vi "initialize ASI stage.vi"(4 "set pcros (um)":cluster{"X":dbl, "Y":dbl, "Z":dbl}, 5 "y range":dbl, 6 "z range":dbl, 7 "x range":dbl, 8 "error in (no error)":errorcluster, 9 "timeout":u32=100, 10 "Baud rate":u32=115200, 11 "VISA resource name":refnum<visa-resource-name>) -> (0 "error out":errorcluster, 3 "ASI stage":T1)   [LabVIEW 2010]
uses:
  stage properties.ctl
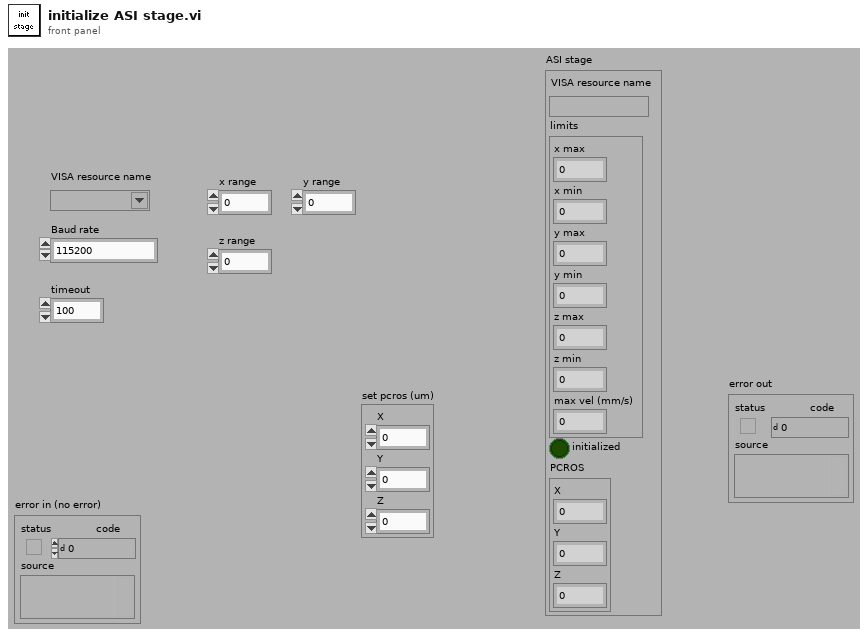
[diagram p1: front panel]
types:
  T1 = typedef "stage properties.ctl" = cluster{"VISA resource name":refnum<visa-resource-name>, "limits":cluster{"x max":dbl, "x min":dbl, "y max":dbl, "y min":dbl, "z max":dbl, "z min":dbl, "max vel (mm/s)":dbl}, "initialized":bool, "PCROS":cluster{"X":dbl, "Y":dbl, "Z":dbl}}
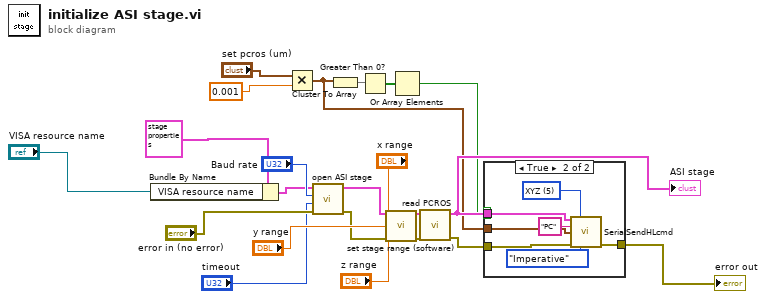
[diagram p0: block diagram]
diagram:
  n1 = Bundle By Name(cluster=T1 {"VISA resource name"="", "limits"={"x max"=0.0, "x min"=0.0, "y max"=0.0, "y min"=0.0, "z max"=0.0, "z min"=0.0, "max vel (mm/s)"=0.0}, "initialized"=FALSE, "PCROS"={"X"=0.0, "Y"=0.0, "Z"=0.0}} ("ASI stage"), "VISA resource name"="VISA resource name") -> (w14:T1)
  n2 = Multiply(x="set pcros (um)", y=0.001 ("x range")) -> (x*y=w5:cluster{"X":dbl, "Y":dbl, "Z":dbl})
  n3 = call "open ASI stage.vi"("error in (no error)"="error in (no error)", "timeout"="timeout", "Baud rate"="Baud rate", "ASI stage"=w14) -> ("error out"=w15:errorcluster, "ASI stage out"=w12:T1)  [unwired: 6 in]
  n4 = Cluster To Array(cluster=w5) -> (array=w4:dbl[])
  n5 = Greater Than 0?(x=w4) -> (x > 0?=w3:bool[])
  n6 = call "set stage range (software).vi"("ASI stage"=w12, "x range"="x range", "y range"="y range", "z range"="z range", "error in (no error)"=w15) -> ("ASI stage out"=w11:T1, "error out"=w10:errorcluster)  [unwired: 9 in]
  n7 = Or Array Elements(Boolean array=w3) -> (logical OR=w2:bool)
  n8 = call "read PCROS.vi"("error in (no error)"=w10, "ASI stage"=w11) -> ("error out"=w8:errorcluster, "ASI stage out"=w9:T1)  [unwired: 8 in]
  "ASI stage" <- w9
  n9 = case shown="True" w2 {
    tunnel: w9 -> [_ w30]
    tunnel: w8 -> [w23 w29]
    tunnel: w5 -> [_ w26]
    tunnel: [w23 w24] -> w1
    frame False {
    }
    frame True {
      w27 = u16 5 items=["No axis", "X", "Y", "Z", "XY", "XYZ"] ("Axis configuration")
      n10 = call "SerialSendHLcmd.vi"("ASI stage"=w30, "Axis configuration"=w27, "Command"="PC", "data in"=w26, "error in (no error)"=w29, "Command type"=enum16{"Query", "Where", "Imperative", "DU Y"}."Imperative") -> ("error out"=w24:errorcluster)  [unwired: 7 in, 2 out]
    }
  }
  "error out" <- w1
